vi "iRobot Navigation Target.vi"() -> ()   [LabVIEW 2015]
uses:
  iRobot Sensors.ctl
  iRobot Navigation State Machine.lvsc/StatechartState.ctl
  iRobot Navigation State Machine.lvsc/State.ctl
  iRobot Navigation State Machine.lvsc/Inputs.ctl
  Accelerometer.ctl
  iRobot/Sensor/Sensor Group 6.ctl
  iRobot/Sensor/Bumps + Wheel Drops.ctl
  iRobot/Sensor/Low-Side Driver + Wheel Overcurrent.ctl
  iRobot/Sensor/Buttons.ctl
  iRobot/Sensor/Charging State.ctl
  iRobot/Sensor/Cargo Bay Digital Inputs.ctl
  iRobot/Sensor/Charging Sources Available.ctl
  iRobot/Sensor/OI Mode.ctl
  iRobot Navigation State Machine.lvsc/CompanionDiagram.vi/61/SC Main.vi
  iRobot Navigation State Machine.lvsc/CompanionDiagram.vi/61/Upd State.vi
  iRobot Navigation State Machine.lvsc/CompanionDiagram.vi/61/Trans Graph0.vi
  iRobot Navigation State Machine.lvsc/CompanionDiagram.vi/61/EnterGraphCore.vi
  <vilib>/myRIO/Common/Instrument Driver Framework/myRIO v1.0/UART/vis/myRIO v1.0 Close UART.vi
  iRobot Navigation State Machine.lvsc/CompanionDiagram.vi/61/Trans Graph1.vi
  iRobot Navigation State Machine.lvsc/CompanionDiagram.vi/61/Trans Graph2.vi
  <vilib>/myRIO/Common/Instrument Driver Framework/myRIO v1.0/myRIO v1.1 Open.vi
  iRobot Navigation State Machine.lvsc/CompanionDiagram.vi
  <vilib>/myRIO/Common/Instrument Driver Framework/Utilities/vis/FPGA Ref Manager.vi
  <vilib>/myRIO/Common/Instrument Driver Framework/myRIO v1.0/myRIO v1.0 Reset FPGA.vi
  <vilib>/myRIO/Common/Instrument Driver Framework/myRIO v1.0/IRQ/vis/myRIO v1.0 IRQ Info FGV.vi
  <vilib>/myRIO/Common/Instrument Driver Framework/myRIO v1.0/IRQ/vis/myRIO v1.0 Timer IRQ Info FGV.vi
  <vilib>/myRIO/Common/Instrument Driver Framework/myRIO v1.0/IRQ/vis/myRIO v1.0 ISR Agent.vi
  iRobot Navigation State Machine.lvsc/Trigger.ctl
  <vilib>/Statechart/Infrastructure/RTStatechart/RunTime SCN.xnode
  iRobot Navigation State Machine.lvsc/Outputs.ctl
  iRobot Navigation State Machine.lvsc
  <vilib>/myRIO/Instrument Drivers/Utilities/Utilities.lvlib
panel:
  in  "stop 2":bool
  in  "Tab Control":T1(tab)
  out "IR Distance(cm)":u16
  out "Right Wheel":i16
  out "Left Wheel":i16
  out "PID output":dbl
  in  "Kd Constant":dbl
  in  "Ki Constant":dbl=30.0
  in  "Kp Constant":dbl=350.0
  out "Current barcode time":dbl
  in  "Barcode Response\nTime Delay":dbl=2.5
  in  "Barcode Time Threshold \n(to measure lenght of each line":dbl=0.45
  in  "Barcode Tape \nSensor Threshold":u16=330
  out "iRobot Sensors (graphical)":T2 {"Right Wheel (mm/s)" scale=-500.0..500.0; "Left Wheel (mm/s)" scale=-500.0..500.0}
  in  "Edge Tape\nSensor Threshold":u16=750
  out "Barcode Array":i32[](array[numeric])
  out "StateData.Speed":i16
  out "Unprocessed Webcam Feed":T4(plugin-control)
  out "Processed Traffic Light":T4(plugin-control)
  out "Processed Obstacles":T4(plugin-control)
  out "Vision Data":T5
  out "Obstacle":bool
  out "Active States":T6
  out "error out":errorcluster
  in  "Wheel Speed (mm/s)":i16(slide)=100 scale=0.0..500.0
  in  "accel smoothing (0-1)":dbl=0.1
  in  "stop":bool
  out "Target Running":bool
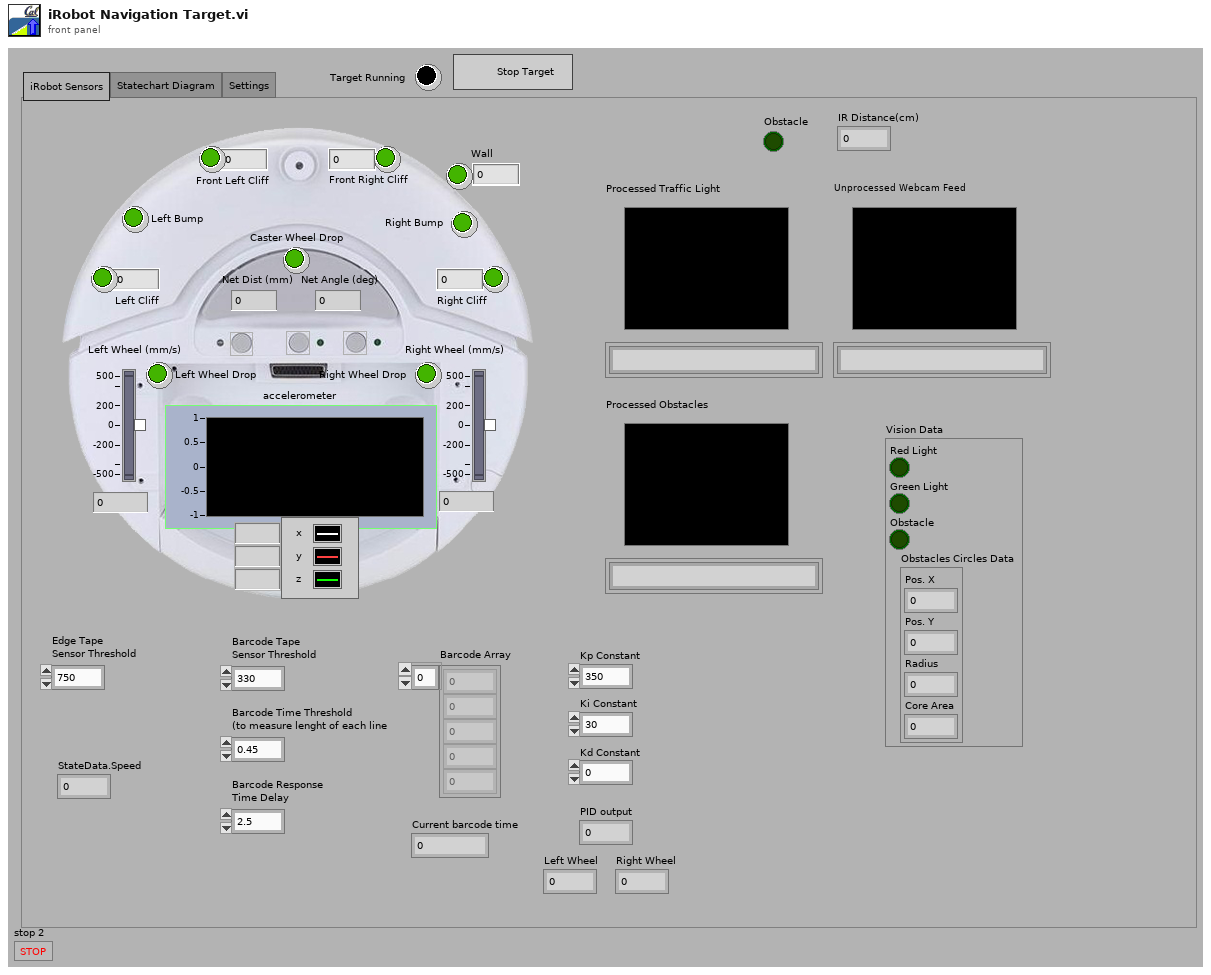
[diagram p1: front panel]
types:
  T1 = enum32{"iRobot Sensors", "Statechart Diagram", "Settings"}
  T2 = typedef "iRobot Sensors.ctl" = cluster{"Caster Wheel Drop":bool, "Left Wheel Drop":bool, "Right Wheel Drop":bool, "Left Bump":bool, "Right Bump":bool, "Left Cliff":bool, "Front Left Cliff":bool, "Front Right Cliff":bool, "Right Cliff":bool, "Wall":bool, "Net Dist (mm)":i32, "Net Angle (deg)":i32, "Wall":u16, "Left Cliff":u16, "Front Left Cliff":u16, "Front Right Cliff":u16, "Right Cliff":u16, "Left Wheel (mm/s)":i16, "Right Wheel (mm/s)":i16, "accelerometer":T3}
  T3 = typedef "Accelerometer.ctl" = cluster{"x axis (g)":dbl, "y axis (g)":dbl, "z axis (g)":dbl}
  T4 = typedef "IMAQ Image.ctl" = refnum<image>
  T5 = cluster{"Red Light":bool, "Green Light":bool, "Obstacle":bool, "Obstacles Circles Data":cluster{"Pos. X":i32, "Pos. Y":i32, "Radius":i32, "Core Area":i32}}
  T6 = typedef "iRobot Navigation State Machine.lvsc/StatechartState.ctl" = T7[]
  T7 = typedef "iRobot Navigation State Machine.lvsc/State.ctl" = enum16{"NI.SC.Initial", "NI.SC.History", "NI.SC.ShallowHistory", "NI.SC.Terminal", "Pause", "Run", "Pause\\Detect Play Button\\Pause;\nWait for\nbutton\nrelease", "Pause\\Detect Play Button\\Unpause;\nwait for\nbutton release", "Pause\\Detect Play Button\\Unpause;\nwait for\nbutton press", "Run\\Detect Obstacles\\Obstacle", "Run\\Detect Obstacles\\Clear line", "Run\\Detect Obstacles\\Object", "Run\\Detect Obstacles\\Red Light", "Run\\Detect Obstacles\\Recover from head on\nedge collision", "Run\\Detect Obstacles\\Check barcode or edge", "Run\\Detect Obstacles\\Right Bumper", "Run\\Detect Obstacles\\Clear the barcode 2", "Run\\Detect Obstacles\\Clear the barcode", "Run\\Detect Obstacles\\Left Bumper", "Run\\Detect Obstacles\\Slow Down", "Run\\Detect Obstacles\\Speed Up", "Run\\Detect Obstacles\\Turn Right", "Run\\Detect Obstacles\\Turn Left", "Run\\Detect Obstacles\\Light", "Run\\Detect Obstacles\\Dark", "Run\\Detect Obstacles\\Straighten Left", "Run\\Detect Obstacles\\Straighten Right", "Run\\Detect Obstacles\\Barcode Drive", "Run\\Detect Obstacles\\Hit Right Boundary /\n Turn Left", "Run\\Detect Obstacles\\Hit Left Boundary / \nTurn Right", "Run\\Detect Obstacles\\Drive"}
  T8 = typedef "iRobot UART Port Type.ctl" = refnum<visa-resource-name>
  T9 = typedef "iRobot Navigation State Machine.lvsc/Inputs.ctl" = cluster{"net distance (mm)":i32, "net angle (deg)":i32, "Max Wheel Speed (mm/s)":i16, "accelerometer":T3, "iRobot Sensors":T10, "Is Simulator?":bool, "Edge Tape Threshold":u16, "Barcode Tape Threshold":u16, "Barcode Time Threshold":dbl, "Barcode Action Time":dbl, "Kp Constant":dbl, "Ki Constant":dbl, "Kd Constant":dbl, "Vision Data":cluster{"Red Light":bool, "Green Light":bool, "Obstacle":bool, "Obstacles Circles Data":cluster{"Pos. X":i32, "Pos. Y":i32, "Radius":i32, "Core Area":i32}}, "IR distance(cm)":u16}
  T10 = typedef "Sensor Group 6.ctl" = cluster{"Bumps + Wheel Drops":T11, "Wall":bool, "Cliff Left":bool, "Cliff Front Left":bool, "Cliff Front Right":bool, "Cliff Right":bool, "Virtual Wall":bool, "Low-Side Driver + Wheel Overcurrent":T12, "Infrared":u8, "Buttons":T13, "Distance (mm)":i32, "Angle (deg)":i32, "Charging State":T14, "Voltage (mV)":u16, "Current (mA)":i16, "Battery Temperature (deg C)":i8, "Battery Charge (mAh)":u16, "Battery Capacity (mAh)":u16, "Wall Signal (0-4095)":u16, "Cliff Left Signal (0-4095)":u16, "Cliff Front Left Signal (0-4095)":u16, "Cliff Front Right Signal (0-4095)":u16, "Cliff Right Signal (0-4095)":u16, "Cargo Bay Digital Inputs":T15, "Cargo Bay Analog Signal (0-1023)":u16, "Charging Sources Available":T16, "OI Mode":T17, "Song Number":u8, "Song Playing":bool, "Number of Stream Packets":u8, "Requested Velocity (mm/s)":i16, "Requested Radius (mm)":i16, "Requested Right Wheel Velocity (mm/s)":i16, "Requested Left Wheel Velocity (mm/s)":i16}
  T11 = typedef "Bumps + Wheel Drops.ctl" = cluster{"Wheeldrop Caster":bool, "Wheeldrop Left":bool, "Wheeldrop Right":bool, "Bump Left":bool, "Bump Right":bool}
  T12 = typedef "Low-Side Driver + Wheel Overcurrent.ctl" = cluster{"Low-Side Driver 0":bool, "Low-Side Driver 1":bool, "Low-Side Driver 2":bool, "Left Wheel":bool, "Right Wheel":bool}
  T13 = typedef "Buttons.ctl" = cluster{"Advance":bool, "Play":bool}
  T14 = typedef "Charging State.ctl" = enum16{"Not Charging", "Reconditioning Charging", "Full Charging", "Trickle Charging", "Waiting", "Charging Fault Condition"}
  T15 = typedef "Cargo Bay Digital Inputs.ctl" = cluster{"Digital Input 0":bool, "Digital Input 1":bool, "Digital Input 2":bool, "Digital Input 3":bool, "Device Detect":bool}
  T16 = typedef "Charging Sources Available.ctl" = cluster{"Internal Charger":bool, "Home Base":bool}
  T17 = typedef "OI Mode.ctl" = enum16{"Off", "Passive", "Safe", "Full"}
  T18 = typedef "iRobot Navigation State Machine.lvsc/Outputs.ctl" = cluster{"Left Wheel Speed (mm/s)":i16, "Right Wheel Speed (mm/s)":i16, "Current time":dbl, "Array":i32[], "PID output":dbl, "Left wheel":i16, "Right wheel":i16, "StateData.Speed":i16, "Obstacle":bool}
  T19 = cluster{"Pos. X":i32, "Pos. Y":i32, "Radius":i32, "Core Area":i32}[]
  T20 = cluster{"Pos. X":i32, "Pos. Y":i32, "Radius":i32, "Core Area":i32}
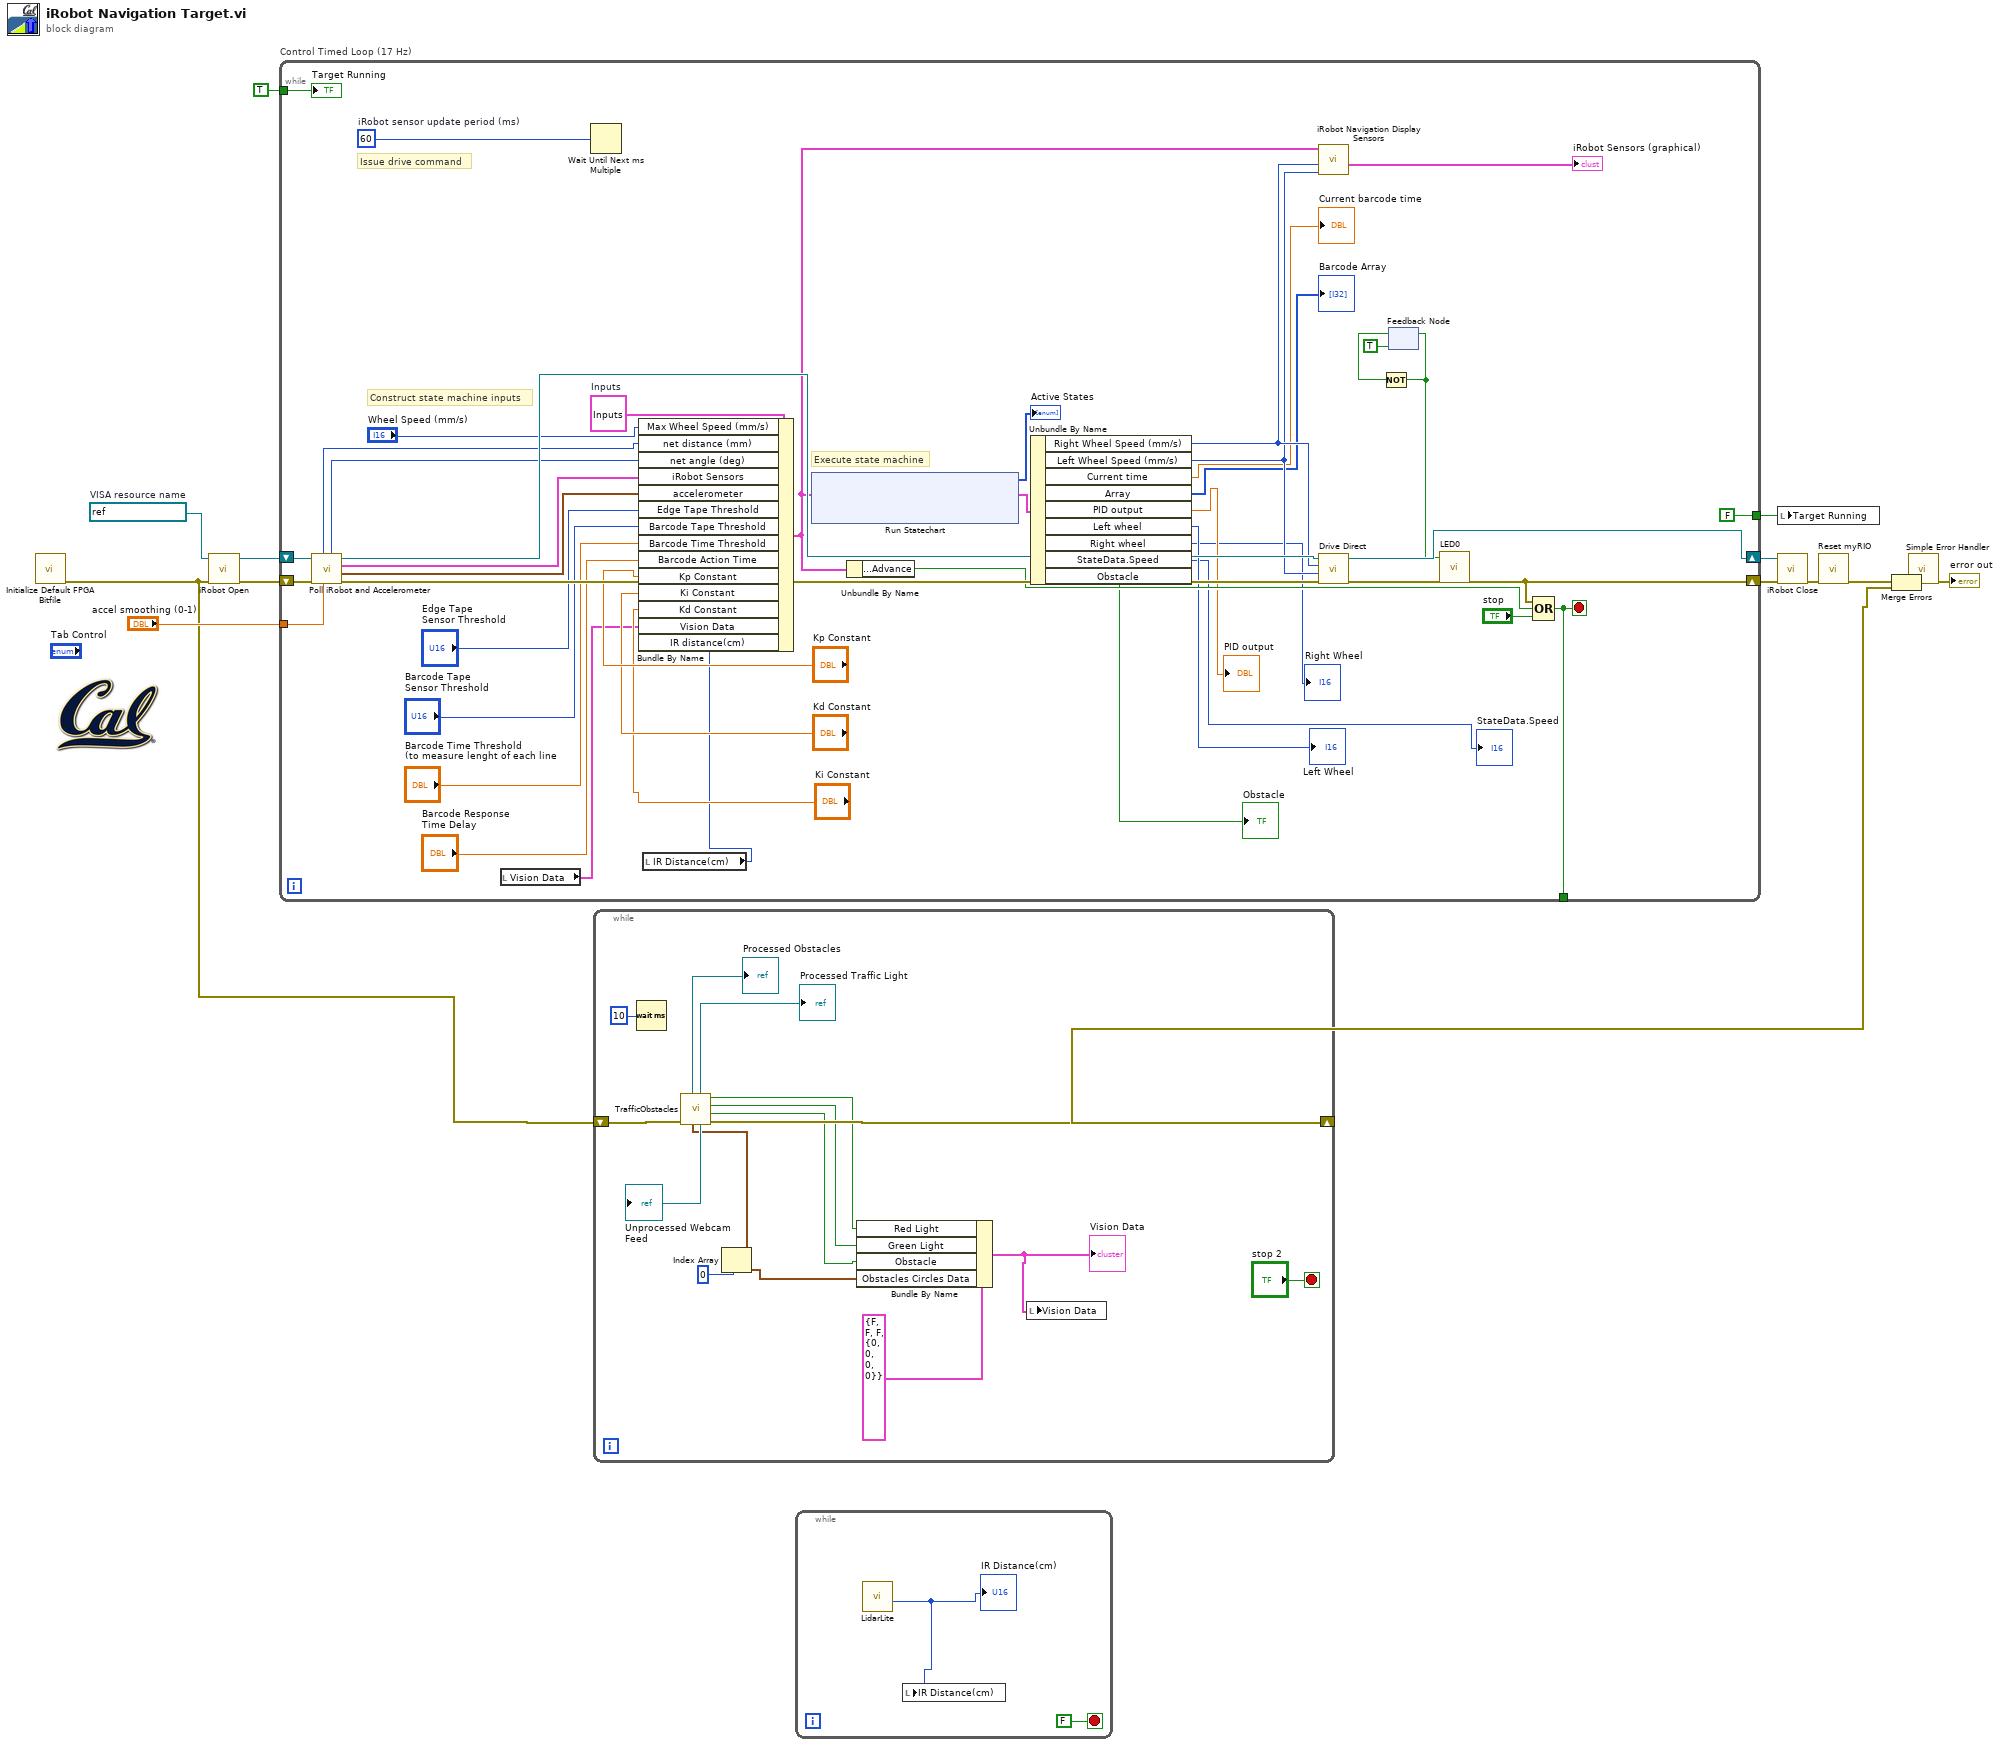
[diagram p0: block diagram]
diagram:
  w8 = refnum<visa-resource-name> "ASRL1::INSTR"  # VISA resource name
  n1 = call <vilib>:"Initialize Default FPGA Bitfile.vi"() -> ("error out"=w2:errorcluster)  [unwired: 11 in]
  n2 = call "iRobot Open.vi"("error in (no error)"=w2, "UART port in"=w8) -> ("error out"=w13:errorcluster, "UART port out"=w12:T8)  [unwired: 8 in]
  n3 = while "Control Timed Loop (17 Hz)" {
    shift-right: [w59] -> w14
    shift-left: w12 -> [w55]
    shift-right: [w42] -> w9
    shift-left: w13 -> [w54]
    tunnel: TRUE ("stop") -> [w48]
    tunnel: [FALSE ("stop")] -> w10
    tunnel: "accel smoothing (0-1)" -> [w34]
    tunnel: [w18] -> _
    stop <- w18 stop-if-true
    w32 = u32 60  # iRobot sensor update period (ms)
    w57 = T9 {"net distance (mm)"=0, "net angle (deg)"=0, "Max Wheel Speed (mm/s)"=0, "accelerometer"={"x axis (g)"=0.0, "y axis (g)"=0.0, "z axis (g)"=0.0}, "iRobot Sensors"={"Bumps + Wheel Drops"={"Wheeldrop Caster"=FALSE, "Wheeldrop Left"=FALSE, "Wheeldrop Right"=FALSE, "Bump Left"=FALSE, "Bump Right"=FALSE}, "Wall"=FALSE, "Cliff Left"=FALSE, "Cliff Front Left"=FALSE, "Cliff Front Right"=FALSE, "Cliff Right"=FALSE, "Virtual Wall"=FALSE, "Low-Side Driver + Wheel Overcurrent"={"Low-Side Driver 0"=FALSE, "Low-Side Driver 1"=FALSE, "Low-Side Driver 2"=FALSE, "Left Wheel"=FALSE, "Right Wheel"=FALSE}, "Infrared"=255, "Buttons"={"Advance"=FALSE, "Play"=FALSE}, "Distance (mm)"=0, "Angle (deg)"=0, "Charging State"=enum."Not Charging", "Voltage (mV)"=0, "Current (mA)"=0, "Battery Temperature (deg C)"=0, "Battery Charge (mAh)"=0, "Battery Capacity (mAh)"=0, "Wall Signal (0-4095)"=0, "Cliff Left Signal (0-4095)"=0, "Cliff Front Left Signal (0-4095)"=0, "Cliff Front Right Signal (0-4095)"=0, "Cliff Right Signal (0-4095)"=0, "Cargo Bay Digital Inputs"={"Digital Input 0"=FALSE, "Digital Input 1"=FALSE, "Digital Input 2"=FALSE, "Digital Input 3"=FALSE, "Device Detect"=FALSE}, "Cargo Bay Analog Signal (0-1023)"=0, "Charging Sources Available"={"Internal Charger"=FALSE, "Home Base"=FALSE}, "OI Mode"=enum."Off", "Song Number"=0, "Song Playing"=FALSE, "Number of Stream Packets"=0, "Requested Velocity (mm/s)"=0, "Requested Radius (mm)"=0, "Requested Right Wheel Velocity (mm/s)"=0, "Requested Left Wheel Velocity (mm/s)"=0}, "Is Simulator?"=FALSE, "Edge Tape Threshold"=0, "Barcode Tape Threshold"=0, "Barcode Time Threshold"=0.0, "Barcode Action Time"=0.0, "Kp Constant"=0.0, "Ki Constant"=0.0, "Kd Constant"=0.0, "Vision Data"={"Red Light"=FALSE, "Green Light"=FALSE, "Obstacle"=FALSE, "Obstacles Circles Data"={"Pos. X"=0, "Pos. Y"=0, "Radius"=0, "Core Area"=0}}, "IR distance(cm)"=0}  # Inputs
    # "Issue drive command"
    # "Execute state machine"
    # "Construct state machine inputs"
    n4 = call "Poll iRobot and Accelerometer.vi"("accel smoothing (0-1)"=w34, "error in"=w54, "UART port in"=w55) -> ("error out"=w53:errorcluster, "Acceleration (g)"=w33:T3, "iRobot SensorGroup6"=w41:T10, "UART port out"=w52:T8, "net angle (deg)"=w50:i32, "net distance (mm)"=w51:i32)  [unwired: 3 in]
    n5 = local read "Vision Data"() -> (w17:T5)
    n6 = Wait Until Next ms Multiple(millisecond multiple=w32) -> ()  [unwired: 1 out]
    n7 = local read "IR Distance(cm)"() -> (w15:u16)
    n8 = Bundle By Name(cluster=w57, "Max Wheel Speed (mm/s)"="Wheel Speed (mm/s)", "net distance (mm)"=w51, "net angle (deg)"=w50, "iRobot Sensors"=w41, "accelerometer"=w33, "Edge Tape Threshold"="Edge Tape\nSensor Threshold", "Barcode Tape Threshold"="Barcode Tape \nSensor Threshold", "Barcode Time Threshold"="Barcode Time Threshold \n(to measure lenght of each line", "Barcode Action Time"="Barcode Response\nTime Delay", "Kp Constant"="Kp Constant", "Ki Constant"="Kd Constant", "Kd Constant"="Ki Constant", "Vision Data"=w17, "IR distance(cm)"=w15) -> (w36:T9)
    n9 = xnode "Run Statechart"("Inputs"=w36) -> ("Outputs"=w58:T18, "Active States"=→"Active States":T6)  [unwired: 2 in, 1 out]
    n10 = Unbundle By Name(w36) -> ("iRobot Sensors.Buttons.Advance"=w35:bool)
    n11 = Unbundle By Name(w58) -> ("Right Wheel Speed (mm/s)"=w39:i16, "Left Wheel Speed (mm/s)"=w38:i16, "Current time"=→"Current barcode time":dbl, "Array"=→"Barcode Array":i32[], "PID output"=→"PID output":dbl, "Left wheel"=→"Left Wheel":i16, "Right wheel"=→"Right Wheel":i16, "StateData.Speed"=→"StateData.Speed":i16, "Obstacle"=→"Obstacle":bool)
    n12 = call "iRobot Navigation Display Sensors.vi"("Left Wheel (mm/s)"=w38, "Right Wheel (mm/s)"=w39, "Statechart Inputs"=w36) -> ("iRobot Sensors (graphical)"=→"iRobot Sensors (graphical)":T2)  [unwired: 6 in]
    n13 = call "Drive Direct.vi"("error in"=w53, "Left Wheel Velocity (mm/s)"=w38, "Right Wheel Velocity (mm/s)"=w39, "UART port in"=w52) -> ("error out"=w43:errorcluster, "UART port out"=w59:T8)  [unwired: 6 in]
    n14 = feedback #1(TRUE) -> (w44:bool)
    n15 = Not(x=w44) -> (.not. x?=w45:bool)
    n16 = feedback-in #1(w45) -> ()
    n17 = call "LED0"("LED0"=w45, "error in (no error)"=w43) -> ("error out"=w42:errorcluster)  [unwired: 25 in]
    n18 = Compound Arithmetic op=OR(w42, w35, "stop") -> (w18:bool)
    "Target Running" <- w48
  }
  n19 = while {
    shift-right: [w238] -> w1
    shift-left: w2 -> [w239]
    stop <- "stop 2" stop-if-true
    n20 = Wait (ms)(milliseconds to wait=u32 10) -> ()  [unwired: 1 out]
    n21 = call "TrafficObstacles.vi"("error in"=w239) -> ("error out"=w238:errorcluster, "Obstacle"=w231:bool, "Green Light"=w232:bool, "Red Light"=w233:bool, "Unprocessed Webcam Feed"=→"Unprocessed Webcam Feed":T4, "Processed Traffic Light"=→"Processed Traffic Light":T4, "Obstacle Circles Data"=w229:T19, "Processed Obstacles"=→"Processed Obstacles":T4)  [unwired: 3 in]
    n22 = Index Array(array=w229, index=0) -> (element=w227:T20)
    n23 = Bundle By Name(cluster=T5 {"Red Light"=FALSE, "Green Light"=FALSE, "Obstacle"=FALSE, "Obstacles Circles Data"={"Pos. X"=0, "Pos. Y"=0, "Radius"=0, "Core Area"=0}} ("Vision Data"), "Red Light"=w233, "Green Light"=w232, "Obstacle"=w231, "Obstacles Circles Data"=w227) -> (w226:T5)
    "Vision Data" <- w226
    n24 = local write "Vision Data"(w226) -> ()
  }
  n25 = while {
    stop <- FALSE stop-if-true
    n26 = call "LidarLite.vi"() -> ("Distance (cm)"=w241:u16)  [unwired: 10 in, 1 out]
    "IR Distance(cm)" <- w241
    n27 = local write "IR Distance(cm)"(w241) -> ()
  }
  n28 = local write "Target Running"(w10) -> ()
  n29 = call "iRobot Close.vi"("error in"=w9, "UART port in"=w14) -> ("error out"=w5:errorcluster)  [unwired: 9 in]
  n30 = call <vilib>:"Reset myRIO.vi"("error in (no error)"=w5) -> ("error out"=w4:errorcluster)  [unwired: 10 in]
  n31 = Merge Errors(w4, w1) -> (w3:errorcluster)
  n32 = call <vilib>:"Simple Error Handler.vi"("error in (no error)"=w3) -> ("error out"=→"error out":errorcluster)  [unwired: 4 in, 4 out]
